vi "golden section algorithm.vi"(8 "error in (no error)":errorcluster, 11 "Autofocus in":refnum<class "Autofocus.lvclass">) -> (0 "error out":errorcluster, 3 "Autofocus out":refnum<class "Autofocus.lvclass">)   [LabVIEW 2012, in "Autofocus.lvclass"]
uses:
  Autofocus.lvclass
  Autofocus.lvclass/Autofocus.ctl
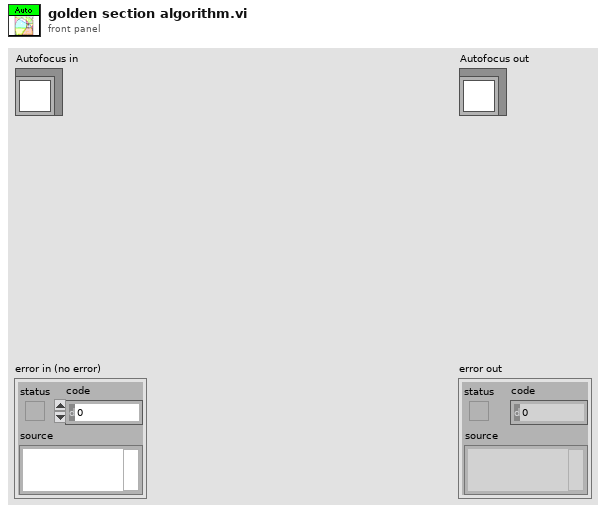
[diagram p1: front panel]
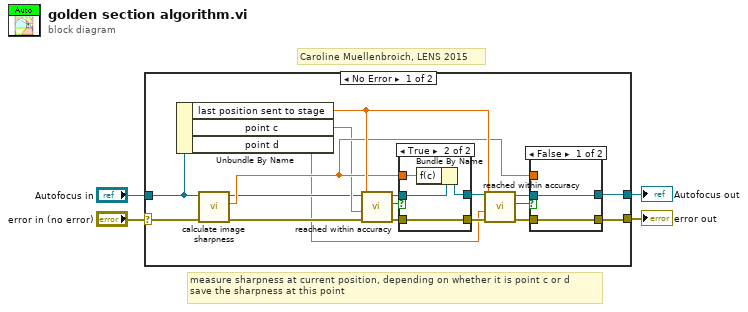
[diagram p0: block diagram]
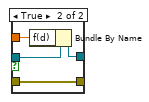
[diagram p2: hidden frame]
diagram:
  # "measure sharpness at current position, depending on whether it is point c or d\nsave the sharpness at this point"
  # "Caroline Muellenbroich, LENS 2015"
  n1 = case shown="No Error" "error in (no error)" {
    selector: "error in (no error)" -> [w9 w36]
    tunnel: [w5 w36] -> w3
    tunnel: [w6 w35] -> w1
    tunnel: "Autofocus in" -> [w8 w35]
    frame No Error {
      n2 = Unbundle By Name(w8) -> ("last position sent to stage"=w22:dbl, "point c"=w12:dbl, "point d"=w7:dbl)
      n3 = call-dynamic "calculate image sharpness.vi"("error in (no error)"=w9, "Autofocus in"=w8) -> ("error out"=w10:errorcluster, "sharpness out"=w16:dbl, "Autofocus out"=w11:refnum<class "Autofocus.lvclass">)  [unwired: 7 in]
      n4 = call-dynamic "reached within accuracy.vi"("error in (no error)"=w10, "destination"=w12, "last position sent to stage"=w22, "Autofocus in"=w11) -> ("error out"=w14:errorcluster, "at destination?"=w13:bool, "Autofocus out"=w15:refnum<class "Autofocus.lvclass">)  [unwired: 5 in]
      n5 = case shown="True" w13 {
        tunnel: w16 -> [_ w34]
        tunnel: w14 -> [w30 w33]
        tunnel: [w30 w33] -> w20
        tunnel: w15 -> [w29 w32]
        tunnel: [w29 w31] -> w21
        frame False {
        }
        frame True {
          n6 = Bundle By Name(cluster=w32, "f(c)"=w34) -> (w31:refnum<class "Autofocus.lvclass">)
        }
      }
      n7 = call-dynamic "reached within accuracy.vi"("error in (no error)"=w20, "destination"=w7, "last position sent to stage"=w22, "Autofocus in"=w21) -> ("error out"=w17:errorcluster, "at destination?"=w18:bool, "Autofocus out"=w19:refnum<class "Autofocus.lvclass">)  [unwired: 5 in]
      n8 = case shown="False" w18 {
        tunnel: w16 -> [_ w28]
        tunnel: w17 -> [w23 w27]
        tunnel: [w23 w27] -> w5
        tunnel: w19 -> [w24 w26]
        tunnel: [w24 w25] -> w6
        frame False {
        }
        frame True {
          n9 = Bundle By Name(cluster=w26, "f(d)"=w28) -> (w25:refnum<class "Autofocus.lvclass">)
        }
      }
    }
    frame Error {
    }
  }
  "error out" <- w3
  "Autofocus out" <- w1
